vi "RobotMap.vi"() -> ()   [LabVIEW 2018]
uses:
  <vilib>/Rock Robotics/SystemInterfaces/AI/FPGA_AIGyroChannel.ctl
  <vilib>/Rock Robotics/SystemInterfaces/DIO/FPGA_DIOChannel.ctl
panel:
  in  "ClimbLimitSwitch":T1=enum."DIO 2"
  in  "Climb Slave":u8=12
  in  "Climb Master":u8=11
  in  "Gyro":T2
  in  "4Bar Limit Switch BottomDIO":dbl
  in  "RightDriveSlave2":u8=10
  in  "LeftDriveSlave2":u8=3
  in  "Cargo Master":dbl=5.0
  in  "Cargo Slave":dbl=6.0
  in  "4BarSlave":u8=7
  in  "4BarMaster":u8=4
  in  "RightDriveSlave1":u8=9
  in  "RightDriveMaster":u8=8
  in  "LeftDriveSlave1":u8=2
  in  "LeftDriveMaster":u8=1
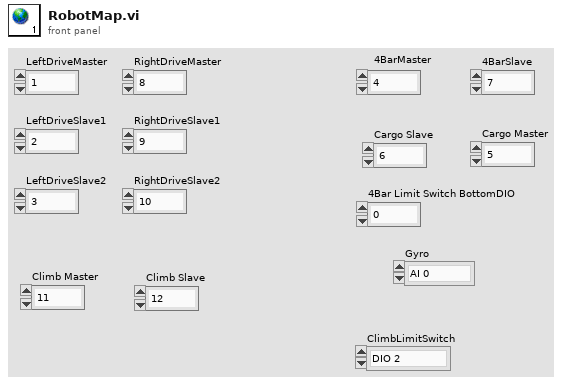
[diagram p1: front panel]
types:
  T1 = typedef "FPGA_DIOChannel.ctl" = enum8{"DIO 0", "DIO 1", "DIO 2", "DIO 3", "DIO 4", "DIO 5", "DIO 6", "DIO 7", "DIO 8", "DIO 9", "DIO MXP 0", "DIO MXP 1", "DIO MXP 2", "DIO MXP 3", "DIO MXP 4", "DIO MXP 5", "DIO MXP 6", "DIO MXP 7", "DIO MXP 8", "DIO MXP 9", "DIO MXP 10", "DIO MXP 11", "DIO MXP 12", "DIO MXP 13", "DIO MXP 14", "DIO MXP 15", "SPI Port CS1", "SPI Port CS2", "SPI Port CS3", "SPI Port MISO", "SPI Port MOSI", "Invalid"}
  T2 = typedef "FPGA_AIGyroChannel.ctl" = enum8{"AI 0", "AI 1", "Invalid"}
diagram:
